vi "draw a line -- complex.vi"(10 "x1":cdb, 11 "x0":cdb) -> (3 "output cluster":cluster{dbl[], dbl[]})   [LabVIEW 2018]
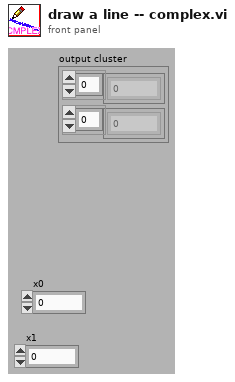
[diagram p1: front panel]
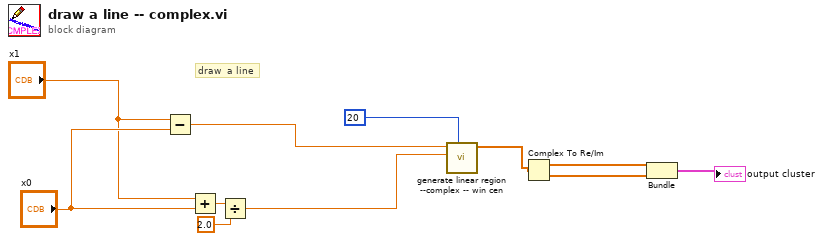
[diagram p0: block diagram]
diagram:
  # "draw  a line"
  n1 = Subtract(x="x1", y="x0") -> (x-y=w5:cdb)
  n2 = Add(x="x1", y="x0") -> (x+y=w11:cdb)
  n3 = Divide(x=w11, y=2.0) -> (x/y=w7:cdb)
  n4 = call "generate linear region --complex -- win cen.vi"("number of  grid points"=20, "center"=w7, "delta"=w5) -> ("real axis"=w4:cdb[])  [unwired: 8 in]
  n5 = Complex To Re/Im(x + iy=w4) -> (x=w3:dbl[], y=w2:dbl[])
  n6 = Bundle(w3, w2) -> (→"output cluster":cluster{dbl[], dbl[]})  [unwired: 1 in]
